vi "RT Driver VI.vi"(6 "Device Clock":string, 9 "Device Inputs FIFO":refnum<k33>, 10 "Device Outputs FIFO":refnum<k33>, 11 "Device Reference":T1 format="%.0x") -> ()   [LabVIEW 2017, in "Exercise 7.1 Engine.lvlib"]
uses:
  Exercise 7.1 Engine.lvlib
  <vilib>/NI Veristand/Custom Device API/Custom Device Item Ref.ctl
  <vilib>/NI Veristand/Custom Device API/Custom Device Channel Type.ctl
  <vilib>/NI Veristand/Custom Device API/Get Item Property (U16).vi
  <vilib>/NI Veristand/Custom Device API/Get Item Property (String).vi
  <vilib>/NI Veristand/Custom Device API/Custom Device API.lvlib
  <vilib>/NI Veristand/Custom Device Tools/Custom Device Utility Library/Custom Device Utility Library.lvlib
panel:
  in  "Initialization Status Notifier":refnum<notifier>
  in  "Status Notifier":refnum<notifier>
  # "Custom Device Template\nv1.0"
  # "Use this template as a starting point for creating a custom device code module. The input controls shown here are specially named controls that the system will use to provide the device loop with data. The controls are not required for the device loop to run. For instance, if the device doesn't produce any output data, then you don't need the Device Outputs FIFO control. If you do use these controls, however, they need to have these exact names to be functional."
  # "The optional status notifier element is used to notify the RT engine of the last state of the custom device, and to indicate the device has completed execution. If this control is not used, a default No Error value is returned to the system when the device finishes execution.\n\nNote: This error state is not checked until the system shuts down. Use an output status channel to send more immediate status values to the system."
  # "This optional input can be used to send the VeriStand Engine the final status of the custom device initalization process. If this control exists on the custom device front panel, the VeriStand Engine will wait for a status update before starting up. If the custom device reports an error, that will abort the execution of the current configuration in the VeriStand Engine.\n\nThis control can be deleted if the custom device does not need to send the initialization status update."
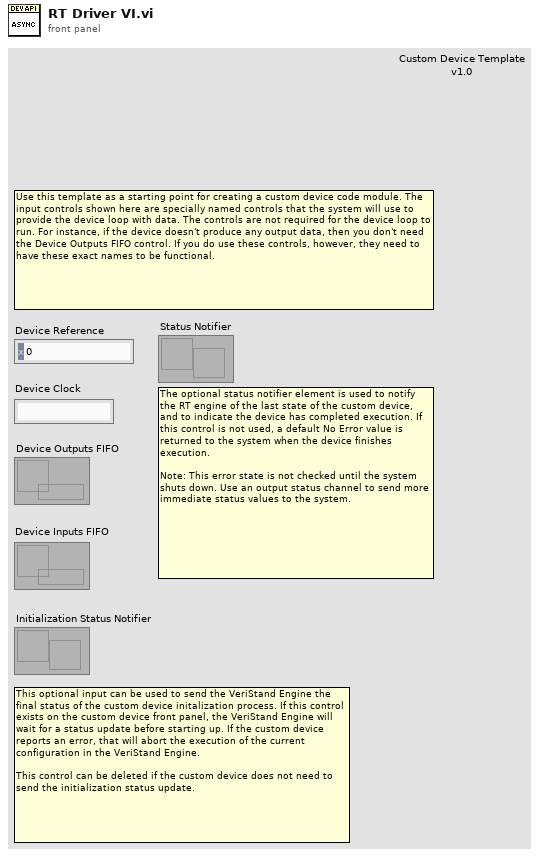
[diagram p1: front panel]
types:
  T1 = typedef "Custom Device API.lvlib/Custom Device Item Ref.ctl" = u64
  T2 = typedef "Custom Device API.lvlib/Custom Device Channel Type.ctl" = enum16{"Input", "Output"}
  T3 = typedef "Custom Device API.lvlib/Custom Device Engine Event Ref.ctl" = refnum<event-registration>
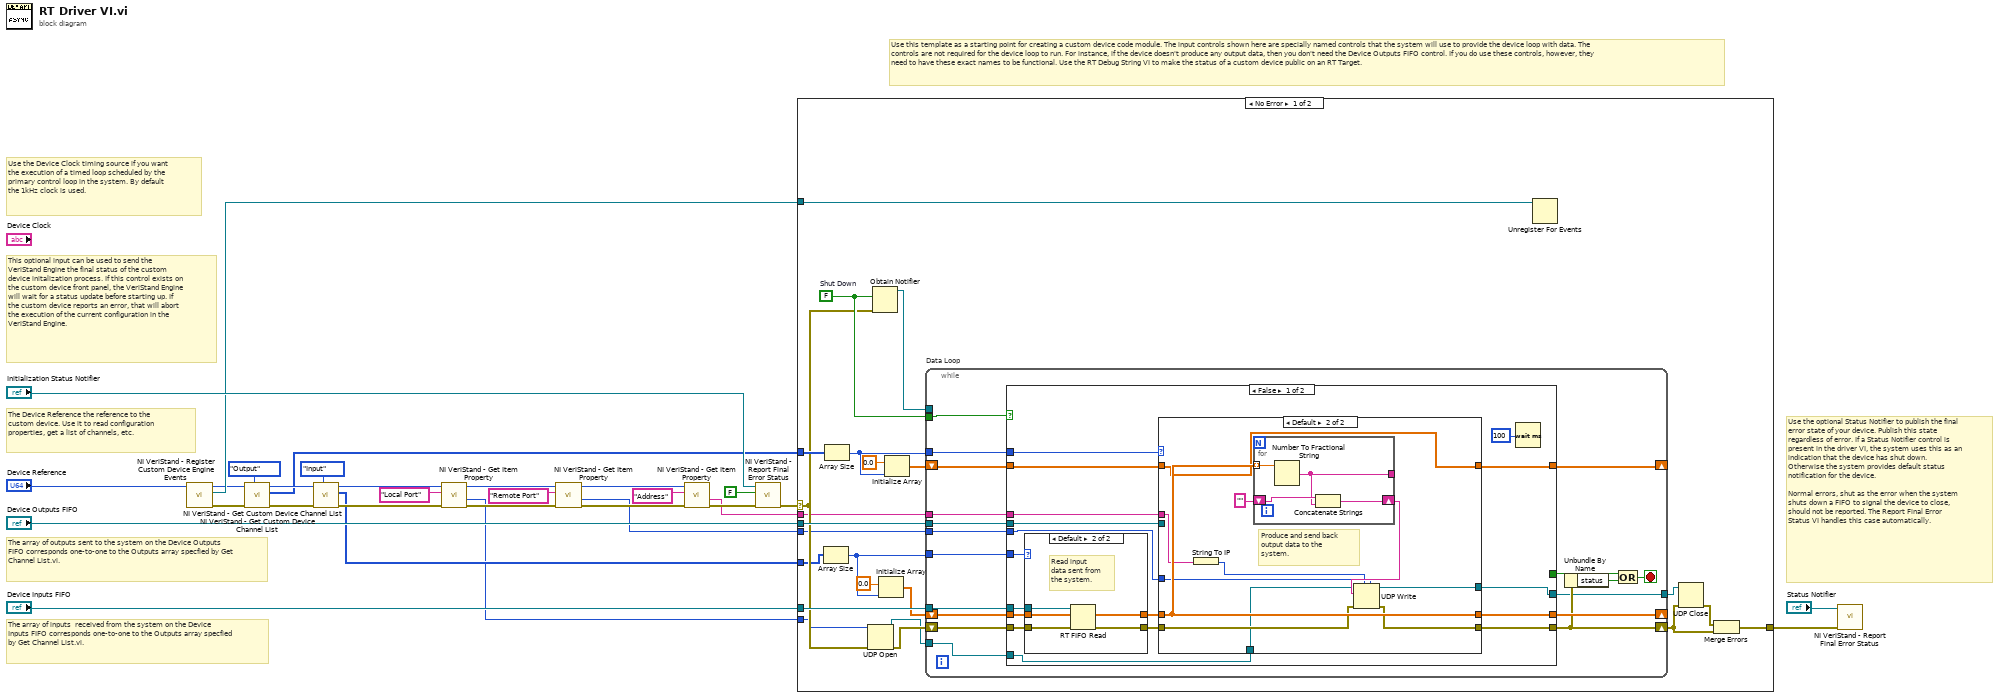
[diagram p0: block diagram]
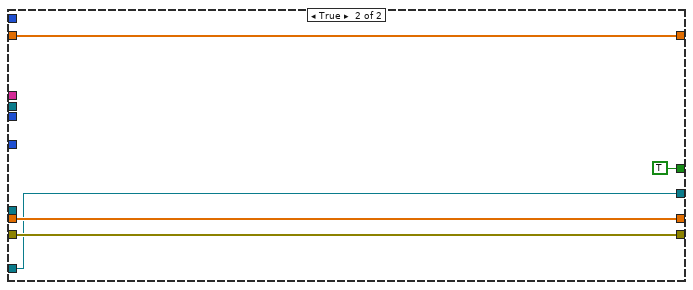
[diagram p4: hidden frame]
diagram:
  # "This optional input can be used to send the VeriStand Engine the final status of the custom device initalization process. If this control exists on the custom device front panel, the VeriStand Engine will wait for a status update before starting up. If the custom device reports an error, that will abort the execution of the current configuration in the VeriStand Engine."
  # "The array of inputs  received from the system on the Device Inputs FIFO corresponds one-to-one to the Outputs array specfied by Get Channel List.vi."
  # "Use the optional Status Notifier to publish the final error state of your device. Publish this state regardless of error. If a Status Notifier control is present in the driver VI, the system uses this as an indication that the device has shut down. Otherwise the system provides default status notification for the device.\n\nNormal errors, shut as the error when the system shuts down a FIFO to signal the device to close, should not be reported. The Report Final Error Status VI handles this case automatically."
  # "The array of outputs sent to the system on the Device Outputs FIFO corresponds one-to-one to the Outputs array specfied by Get Channel List.vi."
  # "The Device Reference the reference to the custom device. Use it to read configuration properties, get a list of channels, etc."
  # "Use the Device Clock timing source if you want the execution of a timed loop scheduled by the primary control loop in the system. By default the 1kHz clock is used."
  # "Use this template as a starting point for creating a custom device code module. The input controls shown here are specially named controls that the system will use to provide the device loop with data. The controls are not required for the device loop to run. For instance, if the device doesn't produce any output data, then you don't need the Device Outputs FIFO control. If you do use these controls, however, they need to have these exact names to be functional. Use the RT Debug String VI to make the status of a custom device public on an RT Target."
  n1 = call <vilib>:"NI VeriStand - Register Custom Device Engine Events.vi"("Device Ref in"="Device Reference") -> ("error out"=w30:errorcluster, "Custom Device Engine Event Ref"=w20:T3, "Device Ref out"=w17:T1)  [unwired: 8 in]
  n2 = call <vilib>:"NI VeriStand - Get Custom Device Channel List.vi"("Channel Type"=Custom_Device_Channel_Type."Output", "error in (no error)"=w30, "Device Ref in"=w17) -> ("error out"=w24:errorcluster, "Specified Channel Ref List"=w22:T1[], "Device Ref out"=w25:T1)  [unwired: 6 out]
  n3 = call <vilib>:"NI VeriStand - Get Custom Device Channel List.vi"("Channel Type"=Custom_Device_Channel_Type."Input", "error in (no error)"=w24, "Device Ref in"=w25) -> ("error out"=w14:errorcluster, "Specified Channel Ref List"=w12:T1[], "Device Ref out"=w13:T1)  [unwired: 6 out]
  n4 = call-poly <vilib>:"NI VeriStand - Get Item Property.vi"("error in (no error)"=w14, "Property Name"="Local Port", "Item Ref in"=w13) -> ("error out"=w11:errorcluster, "Value"=w3:u16, "Item Ref out"=w7:T1)  [unwired: 5 in, 1 out]
  n5 = call-poly <vilib>:"NI VeriStand - Get Item Property.vi"("error in (no error)"=w11, "Property Name"="Remote Port", "Item Ref in"=w7) -> ("error out"=w10:errorcluster, "Value"=w2:u16, "Item Ref out"=w8:T1)  [unwired: 5 in, 1 out]
  n6 = call-poly <vilib>:"NI VeriStand - Get Item Property.vi"("error in (no error)"=w10, "Property Name"="Address", "Item Ref in"=w8) -> ("error out"=w9:errorcluster, "Value"=w1:string)  [unwired: 5 in, 2 out]
  n7 = call <vilib>:"NI VeriStand - Report Final Error Status.vi"("error in (no error)"=w9, "Filter FIFO & Shutdown Errors (T)"=FALSE ("Filter FIFO Errors (T)"), "Status Notifier"="Initialization Status Notifier") -> ("error out"=w16:errorcluster)  [unwired: 8 out]
  n8 = case shown="No Error" w16 {
    selector: w16 -> [w40 w119]
    tunnel: "Device Outputs FIFO" -> [w53 _]
    tunnel: "Device Inputs FIFO" -> [w52 _]
    tunnel: w22 -> [w46 _]
    tunnel: w20 -> [w44 _]
    tunnel: [w42 w119] -> w19
    tunnel: w12 -> [w34 _]
    tunnel: w3 -> [w33 _]
    tunnel: w2 -> [w32 _]
    tunnel: w1 -> [w31 _]
    frame No Error {
      w41 = FALSE  # Shut Down
      n9 = Array Size(array=w34) -> (size(s)=w45:i32)
      n10 = Array Size(array=w46) -> (size(s)=w47:i32)
      n11 = UDP Open(8:w40, 11:w33) -> (port=w38:refnum<k16>, 0:w39:errorcluster)  [unwired: 3 in, 1 out]
      n12 = Obtain Notifier(notification data type=w41, error in (no error)=w40) -> (notifier out=w43:refnum<notifier>)  [unwired: 2 in, 2 out]
      n13 = Initialize Array(0.0 ("element"), w45) -> (w48:dbl[])
      n14 = Initialize Array(0.0 ("element"), w47) -> (w49:dbl[])
      n15 = while "Data Loop" {
        shift-right: [w69] -> _
        shift-left: w48 -> [w70]
        shift-right: [w62] -> w37
        shift-left: w39 -> [w71]
        shift-right: [w67] -> _
        shift-left: w49 -> [w68]
        tunnel: w47 -> [w64]
        tunnel: w53 -> [w66]
        tunnel: w52 -> [w65]
        tunnel: w45 -> [w63]
        tunnel: w43 -> [_]
        tunnel: w41 -> [w58]
        tunnel: w38 -> [w57]
        tunnel: [w56] -> w35
        tunnel: w32 -> [w55]
        tunnel: w31 -> [w54]
        stop <- w59 stop-if-true
        n16 = case shown="False" w58 {
          tunnel: w71 -> [w88 w117]
          tunnel: w70 -> [w87 w118]
          tunnel: [w86 w118] -> w69
          tunnel: w68 -> [w85 w116]
          tunnel: [w84 w116] -> w67
          tunnel: w66 -> [w83 _]
          tunnel: w65 -> [w82 _]
          tunnel: w64 -> [w81 _]
          tunnel: w63 -> [w80 _]
          tunnel: [w77 w117] -> w62
          tunnel: [_ TRUE] -> w60
          tunnel: w57 -> [w75 w114]
          tunnel: [w74 w114] -> w56
          tunnel: w55 -> [w73 _]
          tunnel: w54 -> [w72 _]
          frame False {
            n17 = case shown="Default" w80 {
              tunnel: w82 -> [_ w113]
              tunnel: w87 -> [w108 w112]
              tunnel: [w108 w111] -> w79
              tunnel: [w107 w110] -> w78
              tunnel: w88 -> [w107 w109]
              frame 0 {
                # "No inputs to read\nfrom system. Inputs FIFO not created in this case, so don't write to it."
              }
              frame Default {
                # "Read input data sent from the system."
                n18 = RT FIFO Read(0:w113, 1:w112, 3:w109) -> (9:w111:dbl[], 11:w110:errorcluster)  [unwired: 4 out]
              }
            }
            n19 = case shown="Default" w81 {
              tunnel: w83 -> [_ _]
              tunnel: w85 -> [w91 w94]
              tunnel: w79 -> [w90 w102]
              tunnel: w78 -> [w89 w101]
              tunnel: [w89 w100] -> w77
              tunnel: [w91 w94] -> w84
              tunnel: [w90 w102] -> w86
              tunnel: w75 -> [_ w97]
              tunnel: [_ w96] -> w74
              tunnel: w73 -> [_ w95]
              tunnel: w72 -> [_ w93]
              frame 0 {
                # "No outputs to write to system. The Device Outputs FIFO is never created in this case, so don't write to it."
              }
              frame Default {
                # "Produce and send back output data to the system."
                n20 = String To IP(1:w93) -> (0:w92:u32)
                n21 = for {
                  tunnel: w102 -> [w106] mode=indexing
                  tunnel: [w103] -> _
                  shift-right: [w105] -> w99
                  shift-left: "" -> [w104]
                  n22 = Number To Fractional String(number=w106) -> (F-format string=w103:string)  [unwired: 3 in]
                  n23 = Concatenate Strings(w104, w103) -> (w105:string)
                }
                n24 = UDP Write(address=w92, port or service name=w95, connection ID=w97, data in=w99, 8:w101) -> (error out=w100:errorcluster, 3:w96:refnum<k16>)  [unwired: 1 in]
              }
            }
            n25 = Wait (ms)(milliseconds to wait=u32 100) -> ()  [unwired: 1 out]
          }
          frame True {
          }
        }
        n26 = Unbundle By Name(w62) -> ("status"=w61:bool)
        n27 = Compound Arithmetic op=OR(w60, w61) -> (w59:bool)
      }
      n28 = Unregister For Events(event registration refnum=w44) -> ()  [unwired: 1 in, 1 out]
      n29 = UDP Close(connection ID=w35, 8:w37) -> (error out=w36:errorcluster)  [unwired: 1 out]
      n30 = Merge Errors(w36, w37) -> (w42:errorcluster)
    }
    frame Error {
    }
  }
  n31 = call <vilib>:"NI VeriStand - Report Final Error Status.vi"("error in (no error)"=w19, "Status Notifier"="Status Notifier") -> ()  [unwired: 1 in, 9 out]
